vi "Do.vi"(8 "error in (no error)":cluster{"状态":bool, "代码":i32, "源":string} caption="错误输入（无错误）", 10 "操作者输入":refnum<class "Actor.lvclass">, 11 "Go to Manual消息":refnum<class "Go to Manual消息.lvclass">) -> (0 "error out":cluster{"状态":bool, "代码":i32, "源":string} caption="错误输出", 2 "操作者输出":refnum<class "Actor.lvclass">)   [LabVIEW 2014, in "States.lvlib" / "Go to Manual消息.lvclass"]
doc: "本VI通过对操作者调用合适的方法，将消息发送给操作者。"
uses:
  <vilib>/ActorFramework/Actor/Actor.lvclass
  Process State/CoordinatorState.lvclass
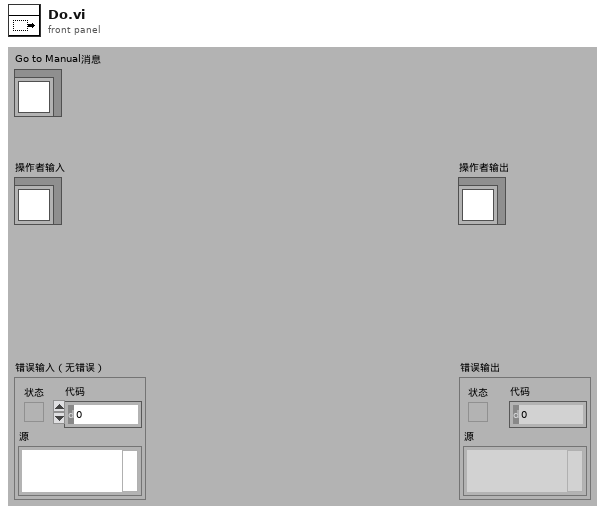
[diagram p1: front panel]
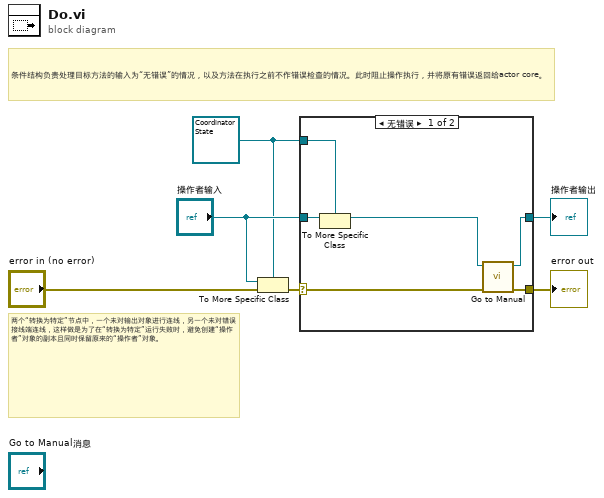
[diagram p0: block diagram]
diagram:
  w1 = refnum<class "CoordinatorState.lvclass"> refnum ("Actor in")
  # "两个“转换为特定”节点中，一个未对输出对象进行连线，另一个未对错误接线端连线，这样做是为了在“转换为特定”运行失败时，避免创建“操作者”对象的副本且同时保留原来的“操作者”对象。"
  # "条件结构负责处理目标方法的输入为“无错误”的情况，以及方法在执行之前不作错误检查的情况。此时阻止操作执行，并将原有错误返回给actor core。"
  n1 = To More Specific Class(target class=w1, reference="操作者输入", error in="error in (no error)") -> (error out=w5:errorcluster)  [unwired: 1 out]
  n2 = case shown="无错误" w5 {
    selector: w5 -> [w10 w14]
    tunnel: [w12 w14] -> w4
    tunnel: [w11 w13] -> w3
    tunnel: "操作者输入" -> [w9 w13]
    tunnel: w1 -> [w8 _]
    frame No Error {
      n3 = To More Specific Class(target class=w8, reference=w9) -> (specific class reference=w7:refnum<class "CoordinatorState.lvclass">)  [unwired: 1 in, 1 out]
      n4 = call-dynamic "Go to Manual.vi"("error in (no error)"=w10, "CommonState in"=w7) -> ("error out"=w12:errorcluster, "CommonState out"=w11:refnum<class "State Actor.lvclass">)  [unwired: 8 in]
    }
    frame Error {
      # "如类型检查失败，则再次将原对象传出。"
    }
  }
  "error out" <- w4
  "操作者输出" <- w3
